vi "Get Number IO.vi"(8 "error in (no error)":errorcluster, 11 "iNumber":i32) -> (0 "error out":errorcluster, 2 "function return":u32, 3 "iNumber out":i32)   [LabVIEW 2014, in "atmcd32d.lvlib"]
doc: "unsigned int WINAPI GetNumberIO(int * iNumber);"
uses:
  atmcd32d.lvlib
  atmcd32d.dll
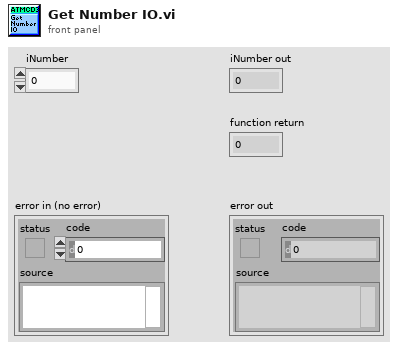
[diagram p1: front panel]
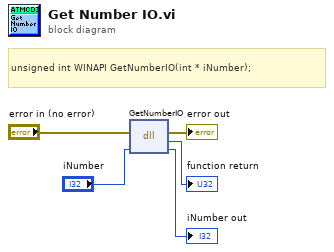
[diagram p0: block diagram]
diagram:
  # "unsigned int WINAPI GetNumberIO(int * iNumber);"
  n1 = dll-call lib="C:/Users/Bakir/Documents/Lambda2-Testing/lib/Andorlib/atmcd32d.*" fn="GetNumberIO"(error in="error in (no error)", "iNumber"="iNumber") -> (error out=→"error out":errorcluster, →"function return":u32, "iNumber"=→"iNumber out":i32)  [unwired: 2 in, 1 out]
